vi "INHERITPUB.constructor.vi"(0 "name":string, 2 "data in":string, 5 "error in(no error)":errorcluster) -> (14 "i ref out":refnum<vi>, 16 "data out":string, 19 "error out":errorcluster)   [LabVIEW 2009]
doc: "This is the constructor of a class.\n\nLicense Agreement for this software:\n\nCopyright (C)\nGesellschaft für Schwerionenforschung, GSI\nPlanckstr. 1\n64291 Darmstadt\nGermany\n\nContact: D.Beck@gsi.de \n\nThis program is free software; you can redistribute it and/or modify it under the terms of the \nGNU General Public License as published by the Free Software Foundation; either version 2 of \nthe license, or (at your option) any later version.\n\nThis program is distributed in the hope that it will be useful, but WITHOUT ANY WARRANTY; \nwithout even the implied warranty of MERCHANTABILITY or FITNESS FOR A PARTICULAR PURPOSE. See the GNU General License for more details (http://www.gnu.org).\n\nGesellschaft für Schwerionenforschung, GSI\nPlanckstr. 1, 64291 Darmstadt, Germany\nFor all questions and ideas contact: M.Richter@gsi.de, H.Brand@gsi.de or D.Beck@gsi.de.\nLast update: 16-JUN-2004"
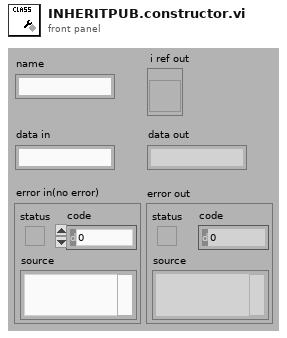
[diagram p1: front panel]
types:
  T1 = enum16{"SetAttribute", "GetAttribute", "CreateAttribute", "DestroyAttribute", "DestroyAllAtributes"}
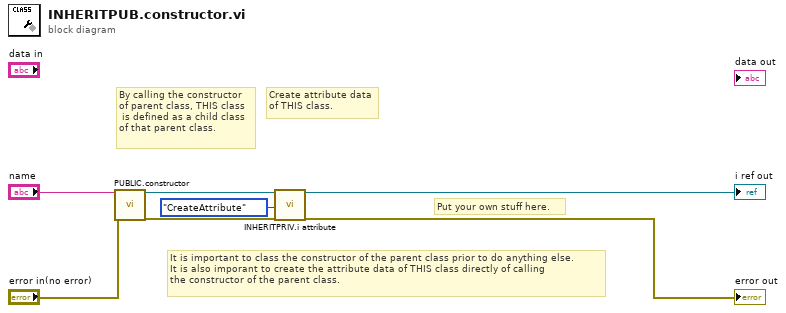
[diagram p0: block diagram]
diagram:
  # "It is important to class the constructor of the parent class prior to do anything else.\nIt is also imporant to create the attribute data of THIS class directly of calling\nthe constructor of the parent class."
  # "Put your own stuff here."
  # "Create attribute data\nof THIS class."
  # "By calling the constructor\nof parent class, THIS class\n is defined as a child class\nof that parent class."
  n1 = call "PUBLIC.constructor.vi"("name"="name", "error in(no error)"="error in(no error)") -> ("i ref out"=w6:refnum<vi>, "error out"=w5:errorcluster)  [unwired: 15 in, 1 out]
  n2 = call "INHERITPRIV.i attribute.vi"("VI Refnum"=w6, "Action"=T1."CreateAttribute", "error in (no error)"=w5) -> ("VI Refnum out"=→"i ref out":refnum<vi>, "error out"=→"error out":errorcluster)  [unwired: 14 in, 1 out]
